vi "TurnPID.vi"(10 "targetValue":dbl) -> ()   [LabVIEW 2016]
uses:
  <vilib>/Rock Robotics/WPI/Utilities/WPI_GetSetVariantRefNum.vi
  Robot Global Data.vi
  <vilib>/addons/control/pid/pid.llb/PID (DBL).vi
  <vilib>/Rock Robotics/WPI/RobotDrive/WPI_RobotDriveArcadeDrive_Standard(NoSaturation).vi
  <vilib>/addons/control/pid/NI_PID_pid.lvlib
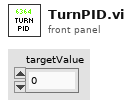
[diagram p1: front panel]
types:
  T1 = typedef "WPI_RobotDriveDevRef.ctl" = cluster{"DevStatus":errorcluster, "Motors[]":T2[], "Square Inputs":bool, "Max Output":dbl}
  T2 = typedef "WPI_MotorControlDeviceRef.ctl" = cluster{"DeviceStatus":errorcluster, "Type":T3, "PWM":cluster{"PWM Channel":T4, "DeadBand":T5}, "CAN":cluster{"Device Number":u8, "SetOutput VI Ref":variant, "GetOutput VI Ref":variant, "Enable VI Ref":variant, "Disable VI Ref":variant, "Data":variant}, "Invert":bool}
  T3 = typedef "WPI_MotorControlType.ctl" = enum16{"PWM", "CAN"}
  T4 = typedef "FPGA_DIOPWMChannel.ctl" = enum8{"PWM 0", "PWM 1", "PWM 2", "PWM 3", "PWM 4", "PWM 5", "PWM 6", "PWM 7", "PWM 8", "PWM 9", "PWM MXP 0", "PWM MXP 1", "PWM MXP 2", "PWM MXP 3", "PWM MXP 4", "PWM MXP 5", "PWM MXP 6", "PWM MXP 7", "PWM MXP 8", "PWM MXP 9", "Invalid"}
  T5 = typedef "WPI_PWMDeadband.ctl" = cluster{"Name":string, "maxPositivePwm":i32, "minPositivePwm":i32, "centerPwm":i32, "maxNegativePwm":i32, "minNegativePwm":i32, "angularRange":u16}
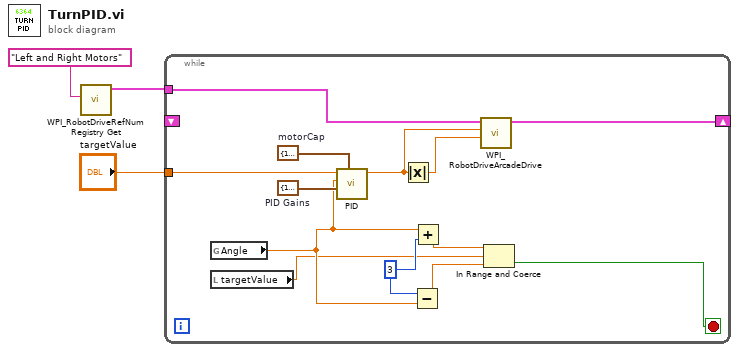
[diagram p0: block diagram]
diagram:
  n1 = call <vilib>:"WPI_RobotDriveRefNum Registry Get.vi"("refnum name"="Left and Right Motors") -> ("RobotDriveDevRef"=w1:T1)  [unwired: 9 in, 1 out]
  n2 = while {
    tunnel: "targetValue" -> [w14]
    tunnel: w1 -> [w7]
    shift-right: [w4] -> _
    shift-left: _ -> [_]
    stop <- w8 stop-if-true
    w13 = 3
    w15 = cluster{dbl, dbl} {1.0, -1.0}  # motorCap
    w16 = cluster{dbl, dbl, dbl} {1.5, 0.0, 6.0}  # PID Gains
    n3 = global read "Robot Global Data.vi" "Angle"() -> (w12:dbl)
    n4 = local read "targetValue"() -> (w9:dbl)
    n5 = call-poly <vilib>:"PID.vi"("output range"=w15, "PID gains"=w16, "process variable"=w12, "setpoint"=w14) -> ("output"=w5:dbl)  [unwired: 6 in, 1 out]
    n6 = Absolute Value(x=w5) -> (abs(x)=w6:dbl)
    n7 = Subtract(x=w13, y=w12) -> (x-y=w10:dbl)
    n8 = Add(x=w12, y=w13) -> (x+y=w11:dbl)
    n9 = call-poly <vilib>:"WPI_RobotDriveArcadeDrive.vi"("Y axis value"=w6, "X axis value"=w5, "RobotDriveDevRef"=w7) -> ("RobotDriveDevRef"=w4:T1)  [unwired: 6 in, 2 out]
    n10 = In Range and Coerce(upper limit=w11, x=w9, lower limit=w10) -> (In Range?=w8:bool)  [unwired: 1 out]
  }
